vi "2B_Tech Serial Data Driver.vi"() -> ()   [LabVIEW 2014]
uses:
  <vilib>/Instr/_visa.llb/VISA Set IO Buffer Mask.ctl
  <vilib>/Instr/_visa.llb/VISA Flush IO Buffer Mask.ctl
  <vilib>/Instr/_visa.llb/VISA Configure Serial Port (Instr).vi
panel:
  out "Data Output":string
  out "return count":u32
  out "Bytes Read":u32
  out "error out 2":errorcluster
  in  "timeout (10sec)":u32=3000
  out "Waveform Chart":u32(graph)
  in  "VISA resource name":refnum<visa-resource-name>="ASRL2::INSTR"
  out "Number of times \nRead time out":u32
  out "Max Time diff":u32
  out "Time diff":u32
  out "Loop count":i32
  out "error out":errorcluster
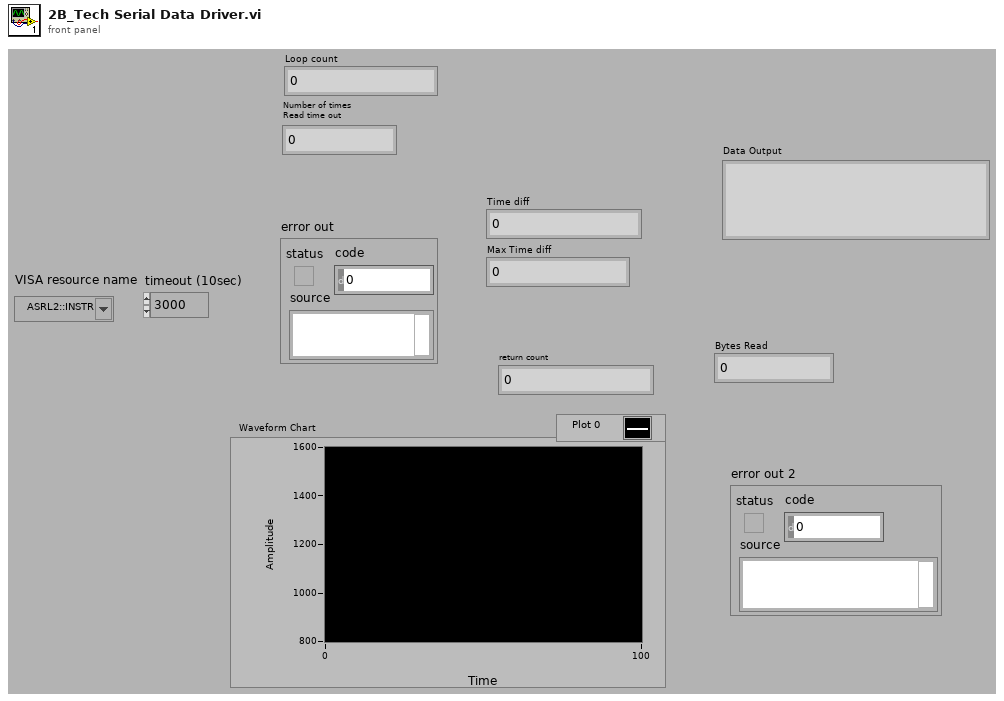
[diagram p1: front panel]
types:
  T1 = typedef "VISA Flush IO Buffer Mask.ctl" = u16
  T2 = typedef "VISA Set IO Buffer Mask.ctl" = u16
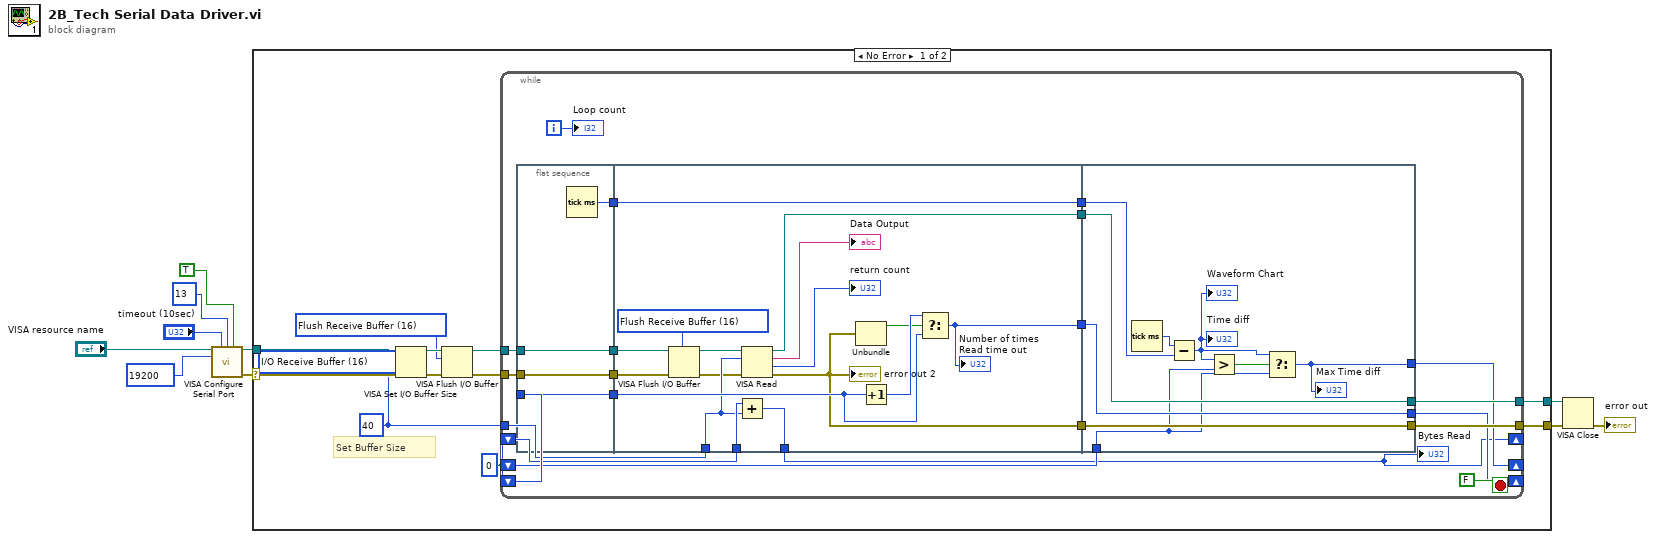
[diagram p0: block diagram]
diagram:
  n1 = call-poly "VISA Configure Serial Port"("VISA resource name"="VISA resource name", "timeout (10sec)"="timeout (10sec)", "termination char\n(0xA = '\\n' = LF)"=u8 13 ("termination char\n(0xA = '\\n' = LF)"), "Enable Termination\nChar (T)"=TRUE ("Enable Termination\nChar (T)"), "baud rate (9600)"=u32 19200) -> ("VISA resource name out"=w10:refnum<visa-resource-name>, "error out"=w6:errorcluster)  [unwired: 9 in]
  n2 = case shown="No Error" w6 {
    selector: w6 -> [w16 w74]
    tunnel: w10 -> [w17 w75]
    tunnel: [w21 w75] -> w9
    tunnel: [w22 w74] -> w8
    frame No Error {
      w11 = u32 40 ("size (4096)")
      w12 = T1 16 items=["Flush Receive Buffer"=16, "Write Transmit Buffer to Device"=32, "Flush Receive Buffer (No I/O)"=64, "Flush Transmit Buffer"=128] ("Mask")
      w13 = T2 16 items=["I/O Receive Buffer"=16, "I/O Transmit Buffer"=32, "I/O Receive and Transmit Buffer"=48] ("Mask")
      w20 = u32 0
      # "Set Buffer Size"
      n3 = VISA Set I/O Buffer Size(VISA resource name=w17, mask (16)=w13, size (4096)=w11, error in (no error)=w16) -> (VISA resource name out=w18:refnum<visa-resource-name>, error out=w19:errorcluster)
      n4 = VISA Flush I/O Buffer(VISA resource name=w18, mask (16)=w12, error in (no error)=w19) -> (VISA resource name out=w14:refnum<visa-resource-name>, error out=w15:errorcluster)
      n5 = while {
        tunnel: w14 -> [w43]
        tunnel: w15 -> [w42]
        tunnel: [w40] -> w22
        shift-right: [w36] -> _
        shift-left: w20 -> [w37]
        shift-right: [w26] -> _
        shift-left: w20 -> [w27]
        tunnel: [w39] -> w21
        shift-right: [w24] -> _
        shift-left: w20 -> [w25]
        tunnel: w11 -> [w23]
        i -> [w38]
        stop <- FALSE stop-if-true
        n6 = flat-sequence {
          tunnel: w37 -> [w45]
          tunnel: w42 -> [w46]
          tunnel: w43 -> [w47]
          tunnel: [w47] -> w35
          tunnel: [w46] -> w34
          tunnel: [w45] -> w33
          tunnel: [w44] -> w28
          tunnel: w35 -> [w52]
          tunnel: w34 -> [w50]
          tunnel: w33 -> [w63]
          tunnel: [w60] -> w32
          tunnel: [w64] -> w31
          tunnel: [w62] -> w30
          tunnel: [w61] -> w29
          tunnel: w28 -> [w61]
          tunnel: w25 -> [w59]
          tunnel: [w58] -> w24
          tunnel: w23 -> [w53]
          tunnel: [w71] -> w36
          tunnel: [w72] -> w39
          tunnel: [w73] -> w40
          tunnel: w32 -> [w73]
          tunnel: w31 -> [w72]
          tunnel: w30 -> [w71]
          tunnel: w29 -> [w67]
          tunnel: w27 -> [w66]
          tunnel: [w65] -> w26
          frame #0 {
            n7 = Tick Count (ms)() -> (millisecond timer value=w44:u32)
          }
          frame #1 {
            w48 = T1 16 items=["Flush Receive Buffer"=16, "Write Transmit Buffer to Device"=32, "Flush Receive Buffer (No I/O)"=64, "Flush Transmit Buffer"=128] ("Mask")
            n8 = VISA Flush I/O Buffer(VISA resource name=w52, mask (16)=w48, error in (no error)=w50) -> (VISA resource name out=w51:refnum<visa-resource-name>, error out=w49:errorcluster)
            n9 = Add(x=w59, y=w53) -> (x+y=w58:u32)
            n10 = VISA Read(VISA resource name=w51, byte count=w53, error in (no error)=w49) -> (VISA resource name out=w64:refnum<visa-resource-name>, read buffer=→"Data Output":string, return count=→"return count":u32, error out=w60:errorcluster)
            "error out 2" <- w60
            n11 = Unbundle(w60) -> ("status"=w56:bool)  [unwired: 2 out]
            n12 = Increment(x=w63) -> (x+1=w57:u32)
            n13 = Select(t=w57, s=w56, f=w63) -> (s? t:f=w62:u32)
            "Number of times \nRead time out" <- w62
          }
          frame #2 {
            n14 = Tick Count (ms)() -> (millisecond timer value=w70:u32)
            n15 = Subtract(x=w70, y=w67) -> (x-y=w69:u32)
            "Time diff" <- w69
            "Waveform Chart" <- w69
            n16 = Greater?(x=w69, y=w66) -> (0:w68:bool)
            n17 = Select(t=w69, s=w68, f=w66) -> (s? t:f=w65:u32)
            "Max Time diff" <- w65
          }
        }
        "Loop count" <- w38
        "Bytes Read" <- w24
      }
    }
    frame Error {
    }
  }
  n18 = VISA Close(VISA resource name=w9, error in (no error)=w8) -> (error out=→"error out":errorcluster)
